vi "9T mag temp-field-chamber wait for.vi"(7 "delay":dbl, 8 "Field":bool, 9 "Chamber":bool, 10 "temp":bool, 11 "输出簇":T1={"initialize"=enum."SR830", "6221"={"6221 Resource"="GPIB0::24::INSTR", "Delta status"=FALSE, "电流|RMS(A)"=0.0}, "SR830+6221"={"source"=0, "Current(A)"=0.0, "阻抗(Ohm)"=0.0, "SR830 1"=FALSE, "SR830 2"=FALSE, "SR830 3"=FALSE, "SR830 4"=FALSE, "VISA 1"="", "VISA 2"="", "VISA 3"="", "VISA 4"="", "Reserve 1"=0, "Reserve 2"=-1, "Reserve 3"=-1, "Reserve 4"=-1, "Sensitivity 1"=-1, "Sensitivity 2"=0, "Sensitivity 3"=-1, "Sensitivity 4"=-1, "量程入 1"=0, "量程入 2"=0, "量程入 3"=0, "量程入 4"=0}, "2400"={"2400"=FALSE, "VISA"="", "Output Level (0)"=1e-05, "Compliance  Level (0.1)"=10.0}, "ch"={"ch"=[], "current"=[], "change?"=[], "holding current\nwhen change ch?"=FALSE}, "Instrument"={"335 Resource"="GPIB0::24::INSTR", "Input (0:A)"=0, "Instrument Type"=enum."SVSM", "quantum design"=refnum, "Heater Output (1:1)"=1, "semaphore"=refnum, "TCP master instance"=refnum, "335 Status"=refnum, "M24C Resource"="GPIB0::24::INSTR", "4G supply"="GPIB0::24::INSTR", "Temp Status 24C"=refnum, "Temp"=refnum, "9T信号"=refnum, "limit"={"Field limit"=0.0, "Field rate limit"=0.0, "Temp limit"=0.0, "Temp low limit"=0.0, "Temp rate limit "=0.0}, "4g supply status"=refnum, "vi路径"="", "325 Resource "="GPIB0::24::INSTR", "Input (0:A) 325"=0, "Input (1;B)"=1}, "Aborting"=refnum, "数据文件"=refnum, "warning"=refnum, "2614B"={"2614B chA"=FALSE, "2614B chB"=FALSE, "VISA"=""}, "33522b"={"33522b resource name"="", "零电压"=0.0, "最大电压"=148.0, "间隔"=4.0, "最小电压"=-48.0, "PZT Scan?"=FALSE}, "gating type"=enum."2614(daul)"} {"Instrument"."Input (1;B)" items=["A", "B"]; "Instrument"."Input (0:A) 325" items=["A", "B"]; "Instrument"."Input (0:A)" items=["A", "B"]; "Instrument"."Heater Output (1:1)" items=["1"=1, "2"=2]; "SR830+6221"."Sensitivity 4" items=["Auto Gain"=-1, "2 nV/fA"=0, "5 nV/fA"=1, "10 nV/fA"=2, "20 nV/fA"=3, "50 nV/fA"=4, "100 nV/fA"=5, "200 nV/fA"=6, "500 nV/fA"=7, "1 uV/pA"=8, "2 uV/pA"=9, "5 uV/pA"=10, "10 uV/pA"=11, "20 uV/pA"=12, "50 uV/pA"=13, "100 uV/pA"=14, "200 uV/pA"=15, "500 uV/pA"=16, "1 mV/nA"=17, "2 mV/nA"=18, "5 mV/nA"=19, "10 mV/nA"=20, "20 mV/nA"=21, "50 mV/nA"=22, "100 mV/nA"=23, "200 mV/nA"=24, "500 mV/mA"=25, "1 V/uA"=26]; "SR830+6221"."Sensitivity 3" items=["Auto Gain"=-1, "2 nV/fA"=0, "5 nV/fA"=1, "10 nV/fA"=2, "20 nV/fA"=3, "50 nV/fA"=4, "100 nV/fA"=5, "200 nV/fA"=6, "500 nV/fA"=7, "1 uV/pA"=8, "2 uV/pA"=9, "5 uV/pA"=10, "10 uV/pA"=11, "20 uV/pA"=12, "50 uV/pA"=13, "100 uV/pA"=14, "200 uV/pA"=15, "500 uV/pA"=16, "1 mV/nA"=17, "2 mV/nA"=18, "5 mV/nA"=19, "10 mV/nA"=20, "20 mV/nA"=21, "50 mV/nA"=22, "100 mV/nA"=23, "200 mV/nA"=24, "500 mV/mA"=25, "1 V/uA"=26]; "SR830+6221"."Sensitivity 1" items=["Auto Gain"=-1, "2 nV/fA"=0, "5 nV/fA"=1, "10 nV/fA"=2, "20 nV/fA"=3, "50 nV/fA"=4, "100 nV/fA"=5, "200 nV/fA"=6, "500 nV/fA"=7, "1 uV/pA"=8, "2 uV/pA"=9, "5 uV/pA"=10, "10 uV/pA"=11, "20 uV/pA"=12, "50 uV/pA"=13, "100 uV/pA"=14, "200 uV/pA"=15, "500 uV/pA"=16, "1 mV/nA"=17, "2 mV/nA"=18, "5 mV/nA"=19, "10 mV/nA"=20, "20 mV/nA"=21, "50 mV/nA"=22, "100 mV/nA"=23, "200 mV/nA"=24, "500 mV/mA"=25, "1 V/uA"=26]; "SR830+6221"."Sensitivity 2" items=["Auto Gain"=-1, "2 nV/fA"=0, "5 nV/fA"=1, "10 nV/fA"=2, "20 nV/fA"=3, "50 nV/fA"=4, "100 nV/fA"=5, "200 nV/fA"=6, "500 nV/fA"=7, "1 uV/pA"=8, "2 uV/pA"=9, "5 uV/pA"=10, "10 uV/pA"=11, "20 uV/pA"=12, "50 uV/pA"=13, "100 uV/pA"=14, "200 uV/pA"=15, "500 uV/pA"=16, "1 mV/nA"=17, "2 mV/nA"=18, "5 mV/nA"=19, "10 mV/nA"=20, "20 mV/nA"=21, "50 mV/nA"=22, "100 mV/nA"=23, "200 mV/nA"=24, "500 mV/mA"=25, "1 V/uA"=26]; "SR830+6221"."Reserve 4" items=["Auto Gain"=-1, "2 nV/fA"=0, "5 nV/fA"=1, "10 nV/fA"=2, "20 nV/fA"=3, "50 nV/fA"=4, "100 nV/fA"=5, "200 nV/fA"=6, "500 nV/fA"=7, "1 uV/pA"=8, "2 uV/pA"=9, "5 uV/pA"=10, "10 uV/pA"=11, "20 uV/pA"=12, "50 uV/pA"=13, "100 uV/pA"=14, "200 uV/pA"=15, "500 uV/pA"=16, "1 mV/nA"=17, "2 mV/nA"=18, "5 mV/nA"=19, "10 mV/nA"=20, "20 mV/nA"=21, "50 mV/nA"=22, "100 mV/nA"=23, "200 mV/nA"=24, "500 mV/mA"=25, "1 V/uA"=26]; "SR830+6221"."Reserve 3" items=["Auto Reserve"=-1, "High Reserve"=0, "Normal"=1, "Low Noise"=2]; "SR830+6221"."Reserve 2" items=["Auto Reserve"=-1, "High Reserve"=0, "Normal"=1, "Low Noise"=2]; "SR830+6221"."Reserve 1" items=["Auto Reserve"=-1, "High Reserve"=0, "Normal"=1, "Low Noise"=2]; "SR830+6221"."source" items=["SR830 1", "SR830 2", "SR830 3", "SR830 4"]}) -> ()   [LabVIEW 2019, in "9T cmag.lvlib"]
uses:
  9T cmag.lvlib
  ctl/config.ctl
  <vilib>/NI/Modbus Library/API/Master/Modbus Master.lvclass
  ctl/initialize.ctl
  ctl/Instrument.ctl
  ctl/Instrument Type.ctl
  lib/QDInstrument.dll
  ctl/335 state.ctl
  ctl/limit.ctl
  ctl/9T mag field stauts.ctl
  ctl/warning.ctl
  ctl/Gating type.ctl
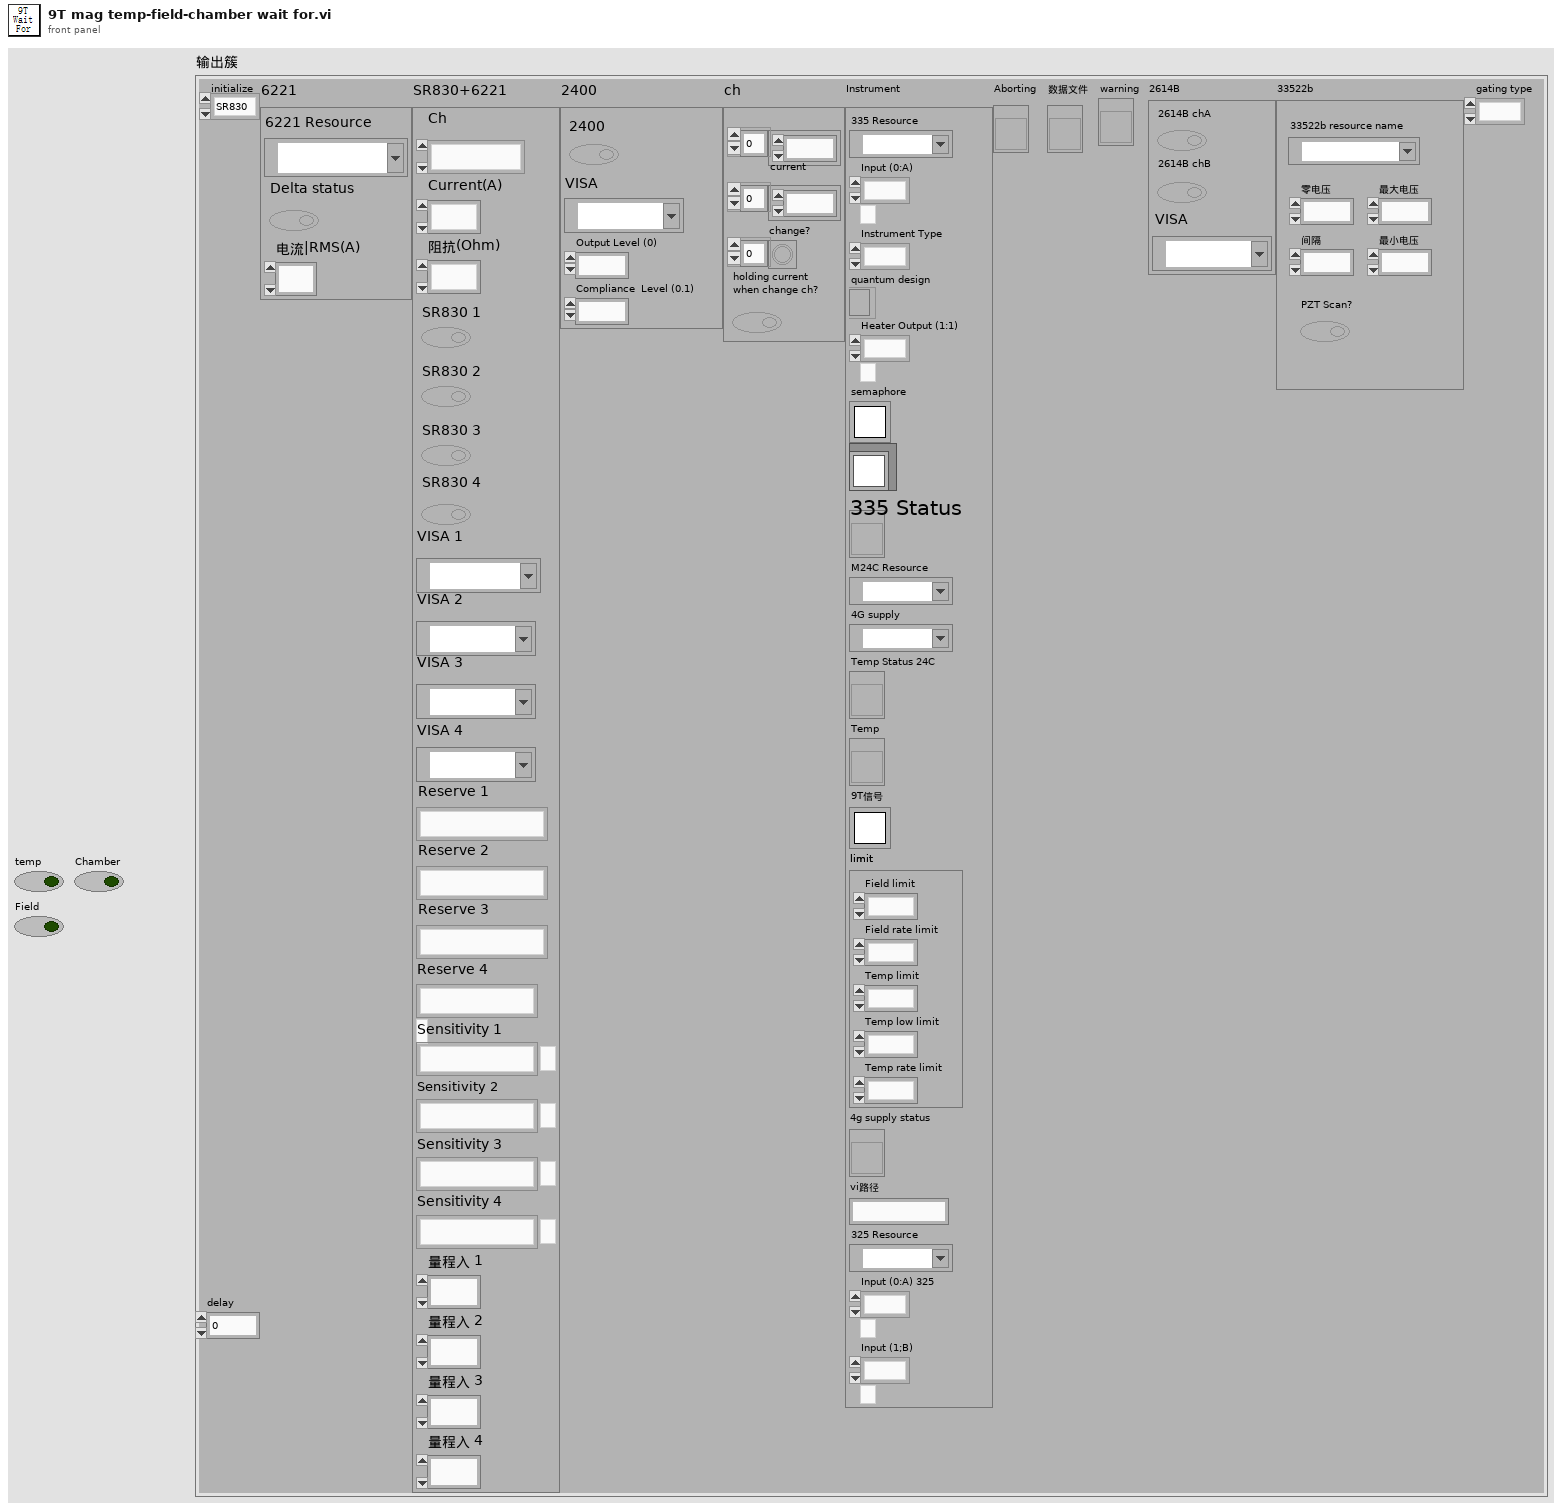
[diagram p1: front panel]
types:
  T1 = typedef "config.ctl" = cluster{"initialize":T2, "6221":cluster{"6221 Resource":refnum<visa-resource-name>, "Delta status":bool, "电流|RMS(A)":dbl}, "SR830+6221":cluster{"source":u16, "Current(A)":dbl, "阻抗(Ohm)":dbl, "SR830 1":bool, "SR830 2":bool, "SR830 3":bool, "SR830 4":bool, "VISA 1":refnum<visa-resource-name>, "VISA 2":refnum<visa-resource-name>, "VISA 3":refnum<visa-resource-name>, "VISA 4":refnum<visa-resource-name>, "Reserve 1":i16, "Reserve 2":i16, "Reserve 3":i16, "Reserve 4":i16, "Sensitivity 1":i16, "Sensitivity 2":i16, "Sensitivity 3":i16, "Sensitivity 4":i16, "量程入 1":i32, "量程入 2":i32, "量程入 3":i32, "量程入 4":i32}, "2400":cluster{"2400":bool, "VISA":refnum<visa-resource-name>, "Output Level (0)":dbl, "Compliance  Level (0.1)":dbl}, "ch":cluster{"ch":i32[], "current":dbl[], "change?":bool[], "holding current\nwhen change ch?":bool}, "Instrument":T3, "Aborting":refnum<vi>, "数据文件":refnum<vi>, "warning":refnum<vi>, "2614B":cluster{"2614B chA":bool, "2614B chB":bool, "VISA":refnum<visa-resource-name>}, "33522b":cluster{"33522b resource name":refnum<visa-resource-name>, "零电压":dbl, "最大电压":dbl, "间隔":dbl, "最小电压":dbl, "PZT Scan?":bool}, "gating type":T7}
  T2 = typedef "initialize.ctl" = enum16{"SR830", "keithley6221-SR830", "Delta", "Delta-tunnelling", "keithley6221-2182-DC", "PZT"}
  T3 = typedef "Instrument.ctl" = cluster{"335 Resource":refnum<visa-resource-name>, "Input (0:A)":u16, "Instrument Type":T4, "quantum design":refnum<k24>, "Heater Output (1:1)":u16, "semaphore":T5, "TCP master instance":refnum<class "Modbus Master.lvclass">, "335 Status":refnum<vi>, "M24C Resource":refnum<visa-resource-name>, "4G supply":refnum<visa-resource-name>, "Temp Status 24C":refnum<vi>, "Temp":refnum<vi>, "9T信号":T5, "limit":T6, "4g supply status":refnum<vi>, "vi路径":string, "325 Resource ":refnum<visa-resource-name>, "Input (0:A) 325":u16, "Input (1;B)":u16}
  T4 = typedef "Instrument Type.ctl" = enum16{"PPMS", "VersaLab", "DynaCool", "SVSM", "PPMS-Rotate", "Lakeshore335", "9T mag"}
  T5 = typedef "Semaphore RefNum" = refnum<k1>
  T6 = typedef "limit.ctl" = cluster{"Field limit":dbl, "Field rate limit":dbl, "Temp limit":dbl, "Temp low limit":dbl, "Temp rate limit ":dbl}
  T7 = typedef "Gating type.ctl" = enum32{"null", "2614(daul)", "2400"}
  T8 = typedef "335 state.ctl" = u16
  T9 = typedef "9T mag field stauts.ctl" = enum16{"unknow", "Stable", "Sweep up", "Sweep down", "Sweep to zero", "Pause"}
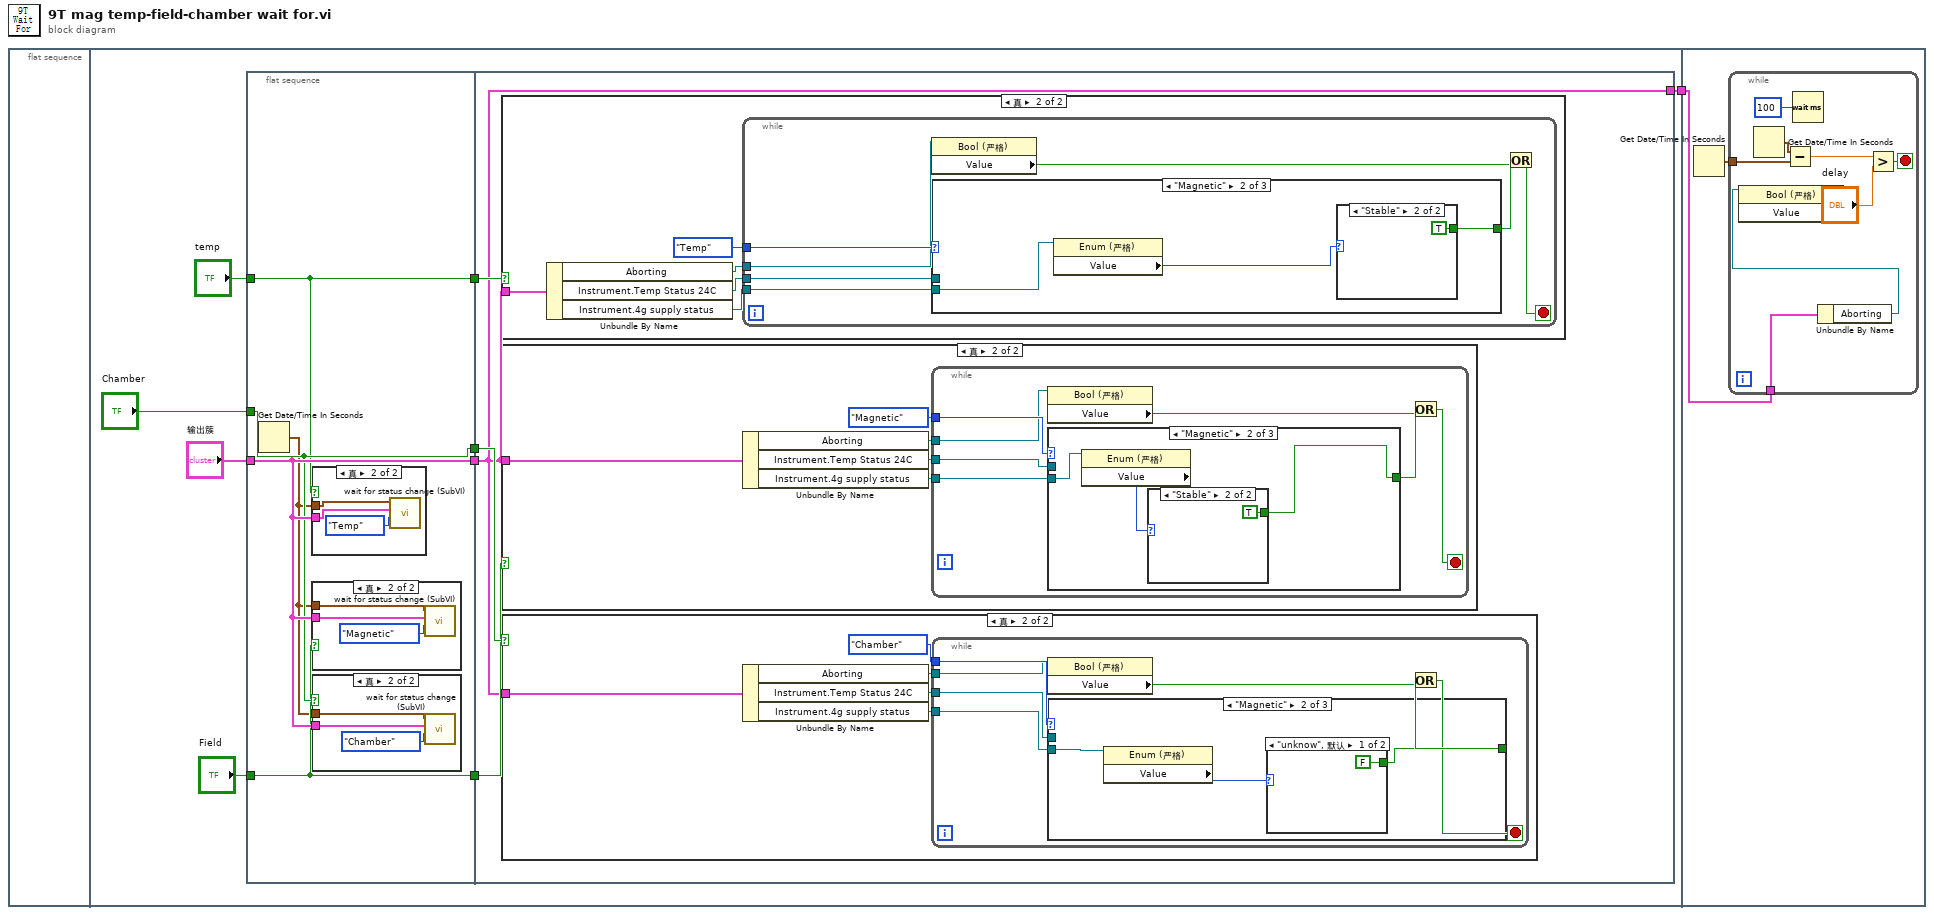
[diagram p0: block diagram]
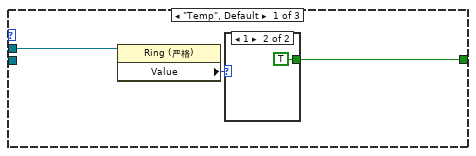
[diagram p6: hidden frame]
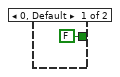
[diagram p7: hidden frame]
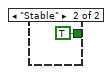
[diagram p8: hidden frame]
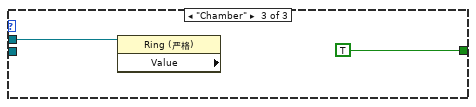
[diagram p9: hidden frame]
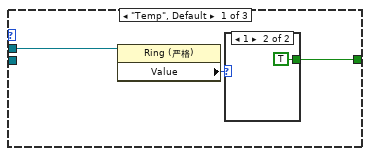
[diagram p11: hidden frame]
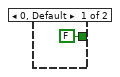
[diagram p12: hidden frame]
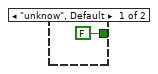
[diagram p13: hidden frame]
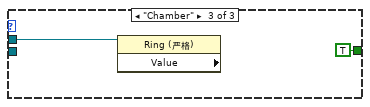
[diagram p14: hidden frame]
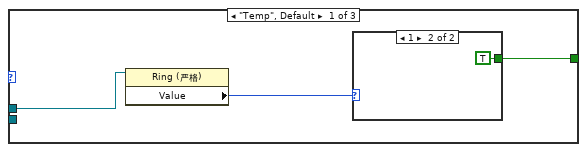
[diagram p16: hidden frame]
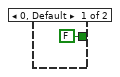
[diagram p17: hidden frame]
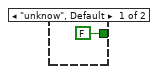
[diagram p18: hidden frame]
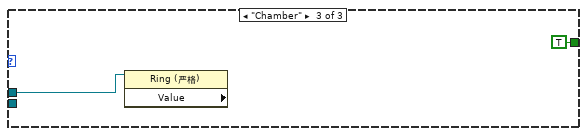
[diagram p19: hidden frame]
diagram:
  n1 = flat-sequence {
    tunnel: [w2] -> w1
    tunnel: w1 -> [w101]
    frame #0 {
    }
    frame #1 {
      n2 = flat-sequence {
        tunnel: "temp" -> [w12]
        tunnel: "Field" -> [w13]
        tunnel: "Chamber" -> [w14]
        tunnel: "输出簇" -> [w15]
        tunnel: [w15] -> w6
        tunnel: [w14] -> w5
        tunnel: [w13] -> w4
        tunnel: [w12] -> w3
        tunnel: w6 -> [w25]
        tunnel: w5 -> [w27]
        tunnel: w4 -> [w26]
        tunnel: w3 -> [w28]
        tunnel: [w25] -> w2
        frame #0 {
          n3 = Get Date/Time In Seconds() -> (seconds since 1Jan1904=w11:timestamp)
          n4 = case shown="真" w12 {
            tunnel: w15 -> [_ w23]
            tunnel: w11 -> [_ w22]
            frame False {
            }
            frame True {
              n5 = call "wait for status change (SubVI).vi"("枚举"=enum16{"Temp", "Magnetic", "Chamber"}."Temp", "输出簇"=w23, "seconds since 1Jan1904"=w22) -> ()  [unwired: 9 in]
            }
          }
          n6 = case shown="真" w13 {
            tunnel: w15 -> [_ w20]
            tunnel: w11 -> [_ w21]
            frame False {
            }
            frame True {
              n7 = call "wait for status change (SubVI).vi"("枚举"=enum16{"Temp", "Magnetic", "Chamber"}."Magnetic", "输出簇"=w20, "seconds since 1Jan1904"=w21) -> ()  [unwired: 9 in]
            }
          }
          n8 = case shown="真" w14 {
            tunnel: w15 -> [_ w17]
            tunnel: w11 -> [_ w18]
            frame False {
            }
            frame True {
              n9 = call "wait for status change (SubVI).vi"("枚举"=enum16{"Temp", "Magnetic", "Chamber"}."Chamber", "输出簇"=w17, "seconds since 1Jan1904"=w18) -> ()  [unwired: 9 in]
            }
          }
        }
        frame #1 {
          n10 = case shown="真" w28 {
            tunnel: w25 -> [_ w78]
            frame False {
            }
            frame True {
              n11 = Unbundle By Name(w78) -> ("Aborting"=w77:refnum<vi>, "Instrument.Temp Status 24C"=w80:refnum<vi>, "Instrument.4g supply status"=w79:refnum<vi>)
              n12 = while {
                tunnel: enum16{"Temp", "Magnetic", "Chamber"}."Temp" ("枚举") -> [w88]
                tunnel: w80 -> [w87]
                tunnel: w79 -> [w86]
                tunnel: w77 -> [w85]
                stop <- w82 stop-if-true
                n13 = property class="Bool (严格)"(reference=w85) -> ("Value"=w83:bool)  [unwired: 1 in, 2 out]
                n14 = case shown="\"Magnetic\"" w88 {
                  tunnel: w87 -> [w90 _ w100]
                  tunnel: w86 -> [_ w96 _]
                  tunnel: [w89 w95 TRUE] -> w84
                  frame "Temp", Default {
                    n15 = property class="Ring (严格)"(reference=w90) -> ("Value"=w91:T8)  [unwired: 1 in, 2 out]
                    n16 = case shown="1" w91 {
                      tunnel: [FALSE TRUE] -> w89
                      frame 0, Default {
                      }
                      frame 1 {
                      }
                    }
                  }
                  frame "Magnetic" {
                    n17 = property class="Enum (严格)"(reference=w96) -> ("Value"=w94:T9)  [unwired: 1 in, 2 out]
                    n18 = case shown="\"Stable\"" w94 {
                      tunnel: [FALSE TRUE] -> w95
                      frame "unknow", Default {
                      }
                      frame "Stable" {
                      }
                    }
                  }
                  frame "Chamber" {
                    n19 = property class="Ring (严格)" props=["Value"](reference=w100) -> ()  [unwired: 1 in, 3 out]
                  }
                }
                n20 = Or(x=w84, y=w83) -> (x .or. y?=w82:bool)
              }
            }
          }
          n21 = case shown="真" w26 {
            tunnel: w25 -> [_ w54]
            frame False {
            }
            frame True {
              n22 = Unbundle By Name(w54) -> ("Aborting"=w53:refnum<vi>, "Instrument.Temp Status 24C"=w56:refnum<vi>, "Instrument.4g supply status"=w55:refnum<vi>)
              n23 = while {
                tunnel: enum16{"Temp", "Magnetic", "Chamber"}."Magnetic" ("枚举") -> [w64]
                tunnel: w56 -> [w63]
                tunnel: w55 -> [w62]
                tunnel: w53 -> [w61]
                stop <- w58 stop-if-true
                n24 = property class="Bool (严格)"(reference=w61) -> ("Value"=w59:bool)  [unwired: 1 in, 2 out]
                n25 = case shown="\"Magnetic\"" w64 {
                  tunnel: w63 -> [w66 _ w76]
                  tunnel: w62 -> [_ w72 _]
                  tunnel: [w65 w70 TRUE] -> w60
                  frame "Temp", Default {
                    n26 = property class="Ring (严格)"(reference=w66) -> ("Value"=w67:T8)  [unwired: 1 in, 2 out]
                    n27 = case shown="1" w67 {
                      tunnel: [FALSE TRUE] -> w65
                      frame 0, Default {
                      }
                      frame 1 {
                      }
                    }
                  }
                  frame "Magnetic" {
                    n28 = property class="Enum (严格)"(reference=w72) -> ("Value"=w71:T9)  [unwired: 1 in, 2 out]
                    n29 = case shown="\"Stable\"" w71 {
                      tunnel: [FALSE TRUE] -> w70
                      frame "unknow", Default {
                      }
                      frame "Stable" {
                      }
                    }
                  }
                  frame "Chamber" {
                    n30 = property class="Ring (严格)" props=["Value"](reference=w76) -> ()  [unwired: 1 in, 3 out]
                  }
                }
                n31 = Or(x=w60, y=w59) -> (x .or. y?=w58:bool)
              }
            }
          }
          n32 = case shown="真" w27 {
            tunnel: w25 -> [_ w30]
            frame False {
            }
            frame True {
              n33 = Unbundle By Name(w30) -> ("Aborting"=w29:refnum<vi>, "Instrument.Temp Status 24C"=w32:refnum<vi>, "Instrument.4g supply status"=w31:refnum<vi>)
              n34 = while {
                tunnel: enum16{"Temp", "Magnetic", "Chamber"}."Chamber" ("枚举") -> [w40]
                tunnel: w32 -> [w39]
                tunnel: w31 -> [w38]
                tunnel: w29 -> [w37]
                stop <- w34 stop-if-true
                n35 = property class="Bool (严格)"(reference=w37) -> ("Value"=w35:bool)  [unwired: 1 in, 2 out]
                n36 = case shown="\"Magnetic\"" w40 {
                  tunnel: w39 -> [w42 _ w52]
                  tunnel: w38 -> [_ w48 _]
                  tunnel: [w41 w46 TRUE] -> w36
                  frame "Temp", Default {
                    n37 = property class="Ring (严格)"(reference=w42) -> ("Value"=w43:T8)  [unwired: 1 in, 2 out]
                    n38 = case shown="1" w43 {
                      tunnel: [FALSE TRUE] -> w41
                      frame 0, Default {
                      }
                      frame 1 {
                      }
                    }
                  }
                  frame "Magnetic" {
                    n39 = property class="Enum (严格)"(reference=w48) -> ("Value"=w47:T9)  [unwired: 1 in, 2 out]
                    n40 = case shown="\"unknow\", 默认" w47 {
                      tunnel: [FALSE TRUE] -> w46
                      frame "unknow", Default {
                      }
                      frame "Stable" {
                      }
                    }
                  }
                  frame "Chamber" {
                    n41 = property class="Ring (严格)" props=["Value"](reference=w52) -> ()  [unwired: 1 in, 3 out]
                  }
                }
                n42 = Or(x=w36, y=w35) -> (x .or. y?=w34:bool)
              }
            }
          }
        }
      }
    }
    frame #2 {
      n43 = Get Date/Time In Seconds() -> (seconds since 1Jan1904=w102:timestamp)
      n44 = while {
        tunnel: w102 -> [w109]
        tunnel: w101 -> [w104]
        stop <- w106 stop-if-true
        n45 = Get Date/Time In Seconds() -> (seconds since 1Jan1904=w110:timestamp)
        n46 = Subtract(x=w110, y=w109) -> (x-y=w108:dbl)
        n47 = Wait (ms)(milliseconds to wait=u32 100) -> ()  [unwired: 1 out]
        n48 = Unbundle By Name(w104) -> ("Aborting"=w103:refnum<vi>)
        n49 = property class="Bool (严格)" props=["Value"](reference=w103) -> ()  [unwired: 1 in, 3 out]
        n50 = Greater?(x=w108, y="delay") -> (0:w106:bool)
      }
    }
  }
